vi "Module - Blank.vi"(8 "error in (no error)":errorcluster) -> (0 "error out":errorcluster)   [LabVIEW 2019]
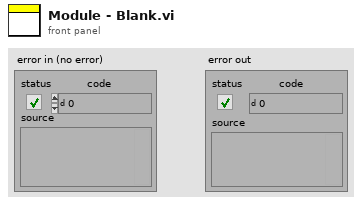
[diagram p1: front panel]
types:
  T1 = enum16{"Init module", "Register for event", "Idle", "Process", "Unregister user event", "Close module"}
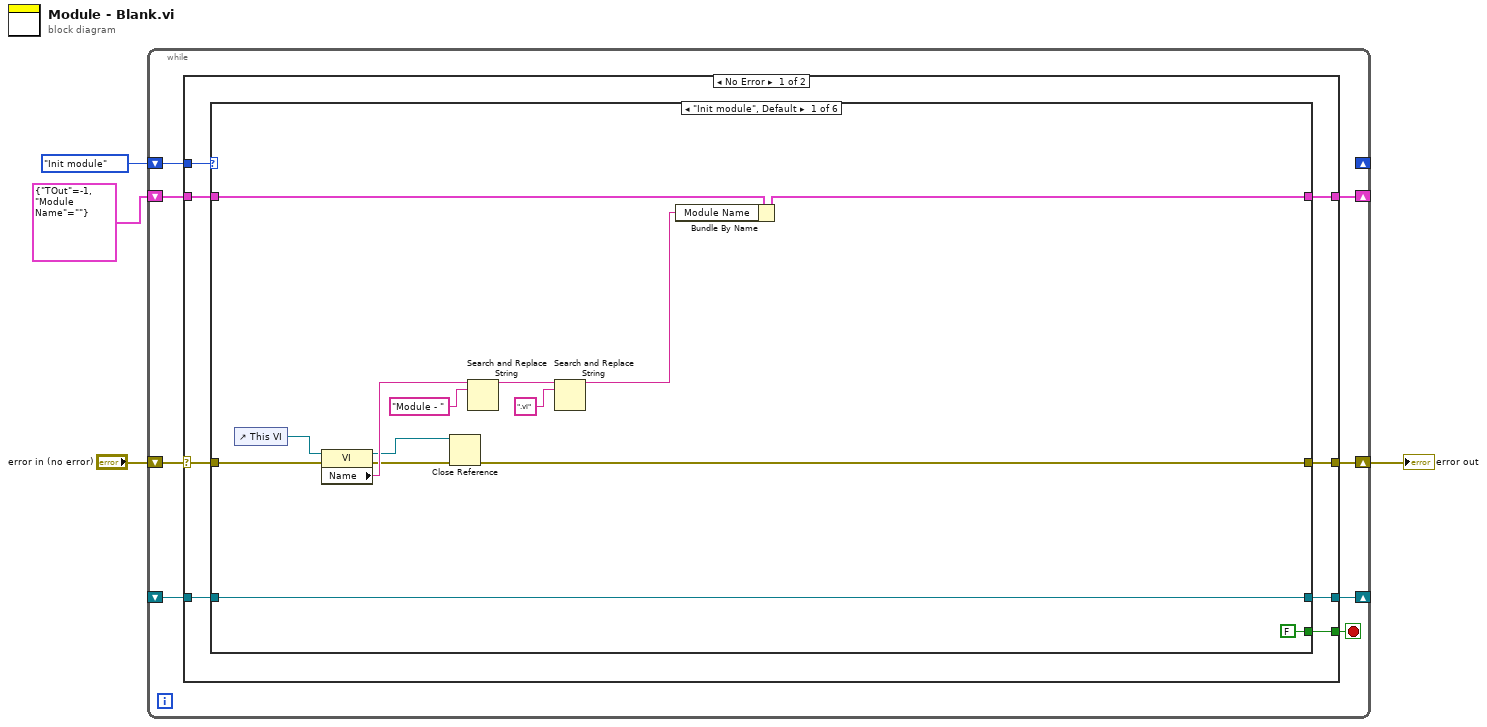
[diagram p0: block diagram]
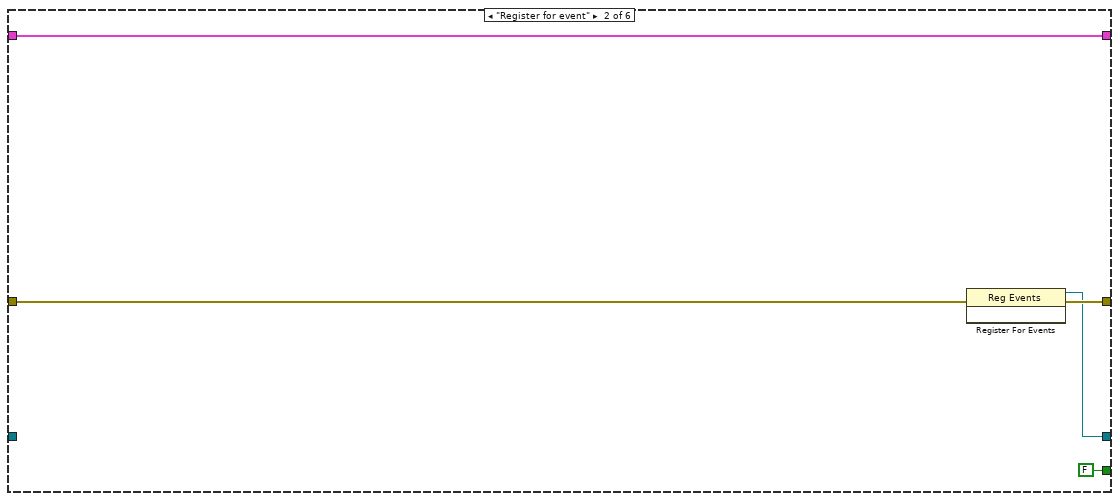
[diagram p2: hidden frame]
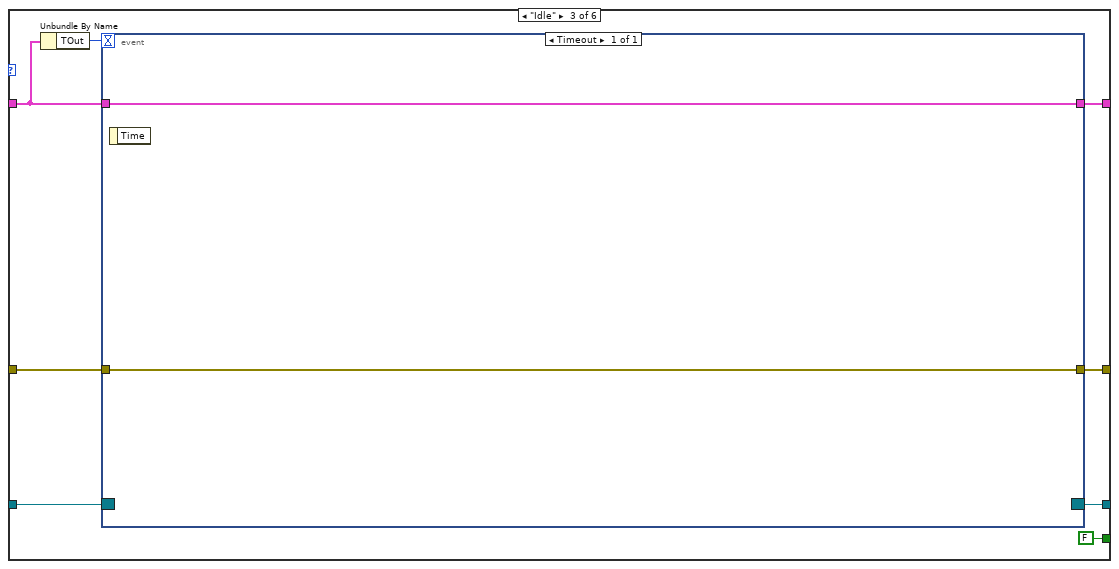
[diagram p3: hidden frame]
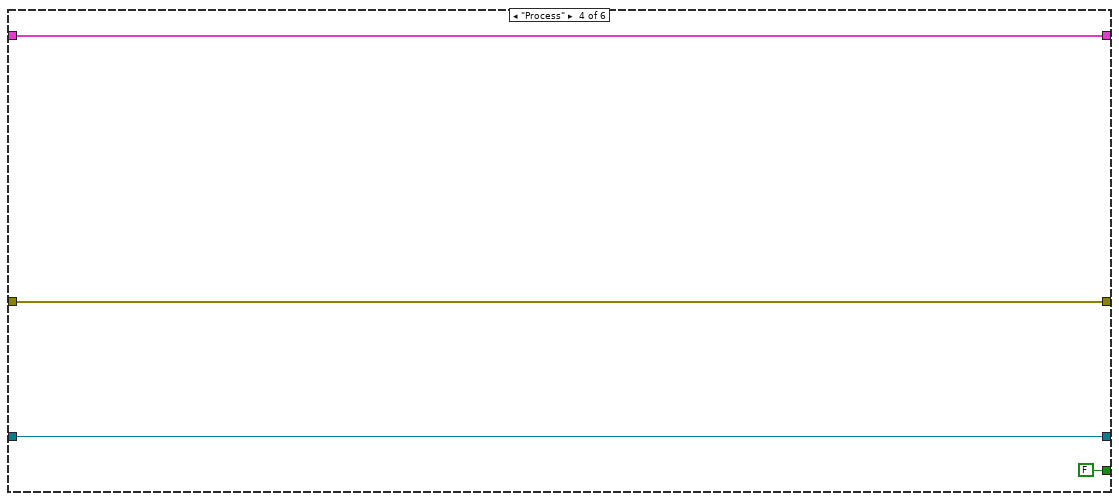
[diagram p4: hidden frame]
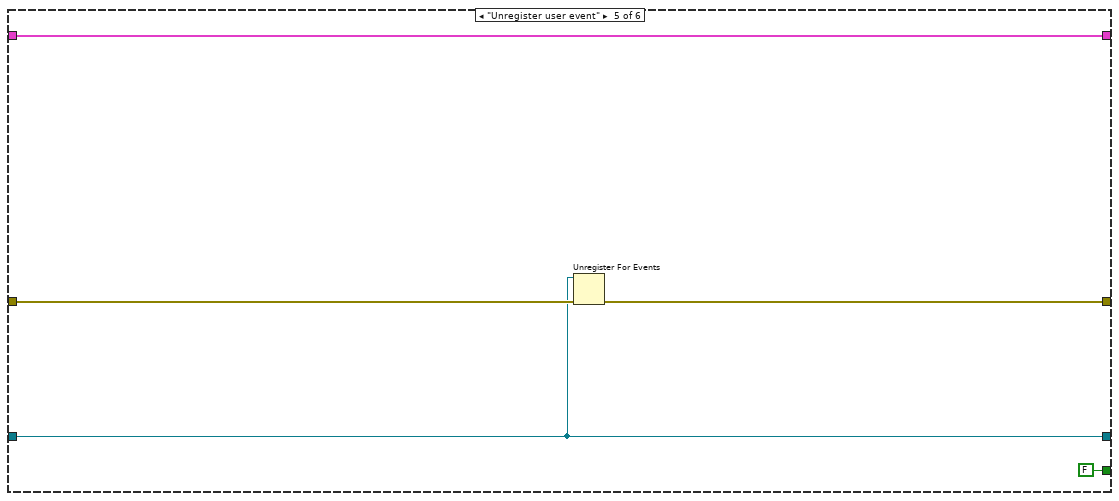
[diagram p5: hidden frame]
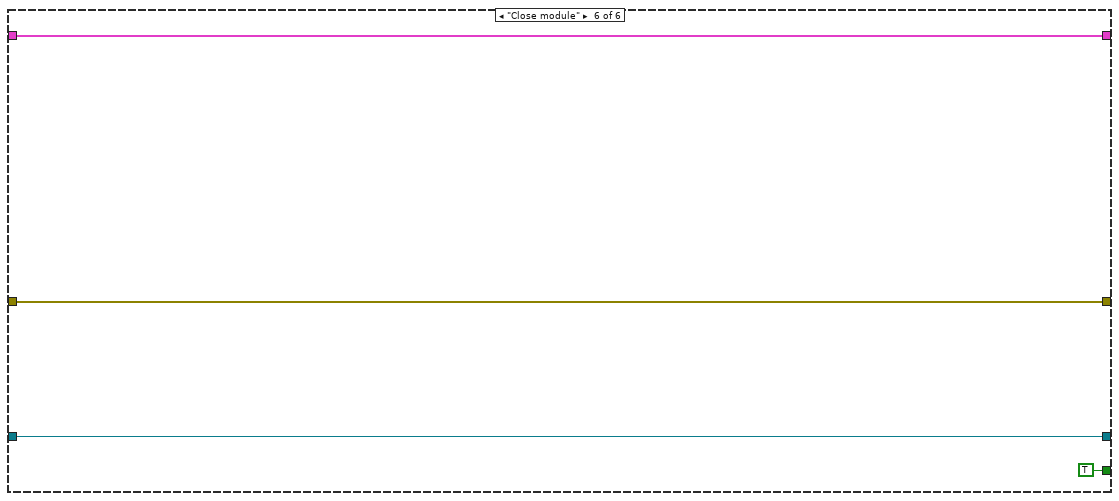
[diagram p6: hidden frame]
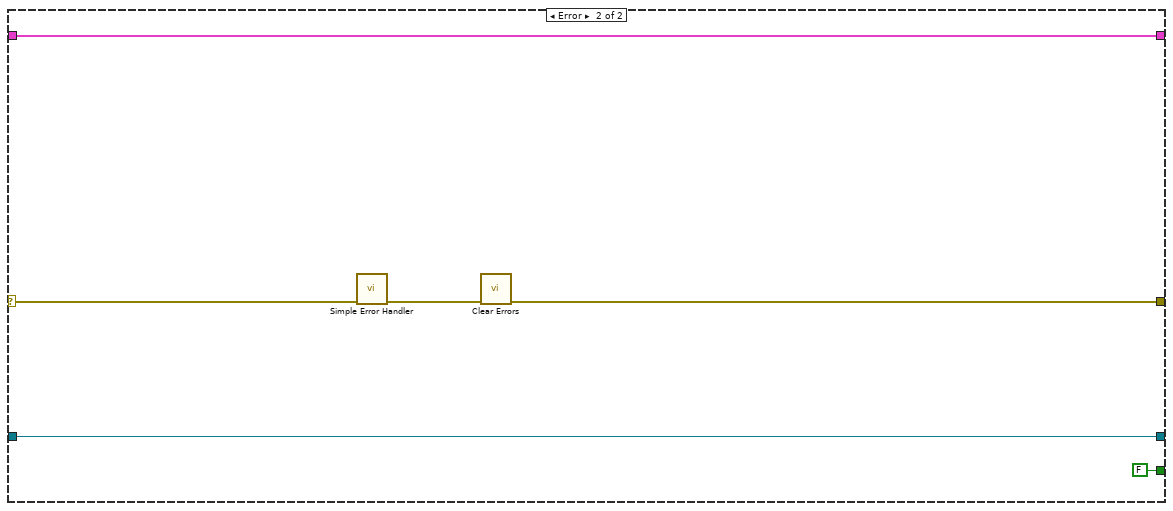
[diagram p7: hidden frame]
diagram:
  n1 = while {
    shift-right: [w8] -> w3
    shift-left: "error in (no error)" -> [w12]
    shift-right: _ -> [_]
    shift-left: T1."Init module" -> [w10]
    shift-right: [w7] -> _
    shift-left: cluster{"TOut":i32, "Module Name":string} {"TOut"=-1, "Module Name"=""} -> [w9]
    shift-right: [w6] -> _
    shift-left: _ -> [w5]
    stop <- w11 stop-if-true
    n2 = case shown="No Error" w12 {
      selector: w12 -> [w20 w66]
      tunnel: [w19 FALSE] -> w11
      tunnel: w10 -> [w18 _]
      tunnel: w9 -> [w17 w63]
      tunnel: [w16 w64] -> w8
      tunnel: [w15 w63] -> w7
      tunnel: [w14 w67] -> w6
      tunnel: w5 -> [w13 w67]
      frame No Error {
        n3 = case shown="\"Init module\", Default" w18 {
          tunnel: w20 -> [w24 w37 w45 w53 w57 w62]
          tunnel: [FALSE FALSE FALSE FALSE FALSE TRUE] -> w19
          tunnel: w17 -> [w33 w35 w42 w52 w58 w61]
          tunnel: [w23 w38 w44 w53 w56 w62] -> w16
          tunnel: [w22 w35 w41 w52 w58 w61] -> w15
          tunnel: [w32 w36 w46 w51 w55 w60] -> w14
          tunnel: w13 -> [w32 _ w47 w51 w55 w60]
          frame "Init module", Default {
            n4 = control-ref of="This VI"() -> (w31:refnum<vi>)
            n5 = property class="VI"(reference=w31, error in=w24) -> (reference out=w25:refnum<vi>, error out=w26:errorcluster, "Name"=w30:string)
            n6 = Close Reference(reference=w25, error in (no error)=w26) -> (error out=w23:errorcluster)
            n7 = Search and Replace String(input string=w30, search string="Module - ") -> (result string=w27:string)  [unwired: 6 in, 3 out]
            n8 = Search and Replace String(input string=w27, search string=".vi") -> (result string=w21:string)  [unwired: 6 in, 3 out]
            n9 = Bundle By Name(cluster=w33, "Module Name"=w21) -> (w22:cluster{"TOut":i32, "Module Name":string})
          }
          frame "Register for event" {
            n10 = register-events(error in=w37) -> (reference out=w36:refnum<event-registration>, error out=w38:errorcluster)  [unwired: 2 in]
          }
          frame "Idle" {
            n11 = Unbundle By Name(w42) -> ("TOut"=w43:i32)
            n12 = event shown="[0] Timeout" {
              selector: w47 -> [_]
              dyn-events: [_] -> w46
              timeout: w43 -> [_]
              tunnel: w45 -> [w49]
              tunnel: [w49] -> w44
              tunnel: w42 -> [w48]
              tunnel: [w48] -> w41
              event Timeout {
                n13 = event-data() -> ()  [unwired: 1 in, 1 out]
              }
            }
          }
          frame "Process" {
          }
          frame "Unregister user event" {
            n14 = Unregister For Events(event registration refnum=w55, error in=w57) -> (error out=w56:errorcluster)
          }
          frame "Close module" {
          }
        }
      }
      frame Error {
        n15 = call <vilib>:"Simple Error Handler.vi"("error in (no error)"=w66) -> ("error out"=w65:errorcluster)  [unwired: 4 in, 4 out]
        n16 = call <vilib>:"Clear Errors.vi"("error in (no error)"=w65) -> ("error out"=w64:errorcluster)  [unwired: 5 in, 1 out]
      }
    }
  }
  "error out" <- w3
